vi "01_dosing.vi"() -> ()   [LabVIEW 2024]
panel:
  out "appended array":bool[](array[boolean])
  in  "Dispense Aliquot (Digital Output (0.4)":bool
  in  "Stop":bool
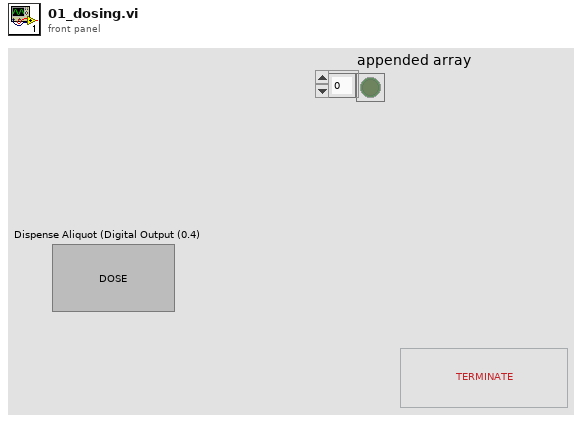
[diagram p1: front panel]
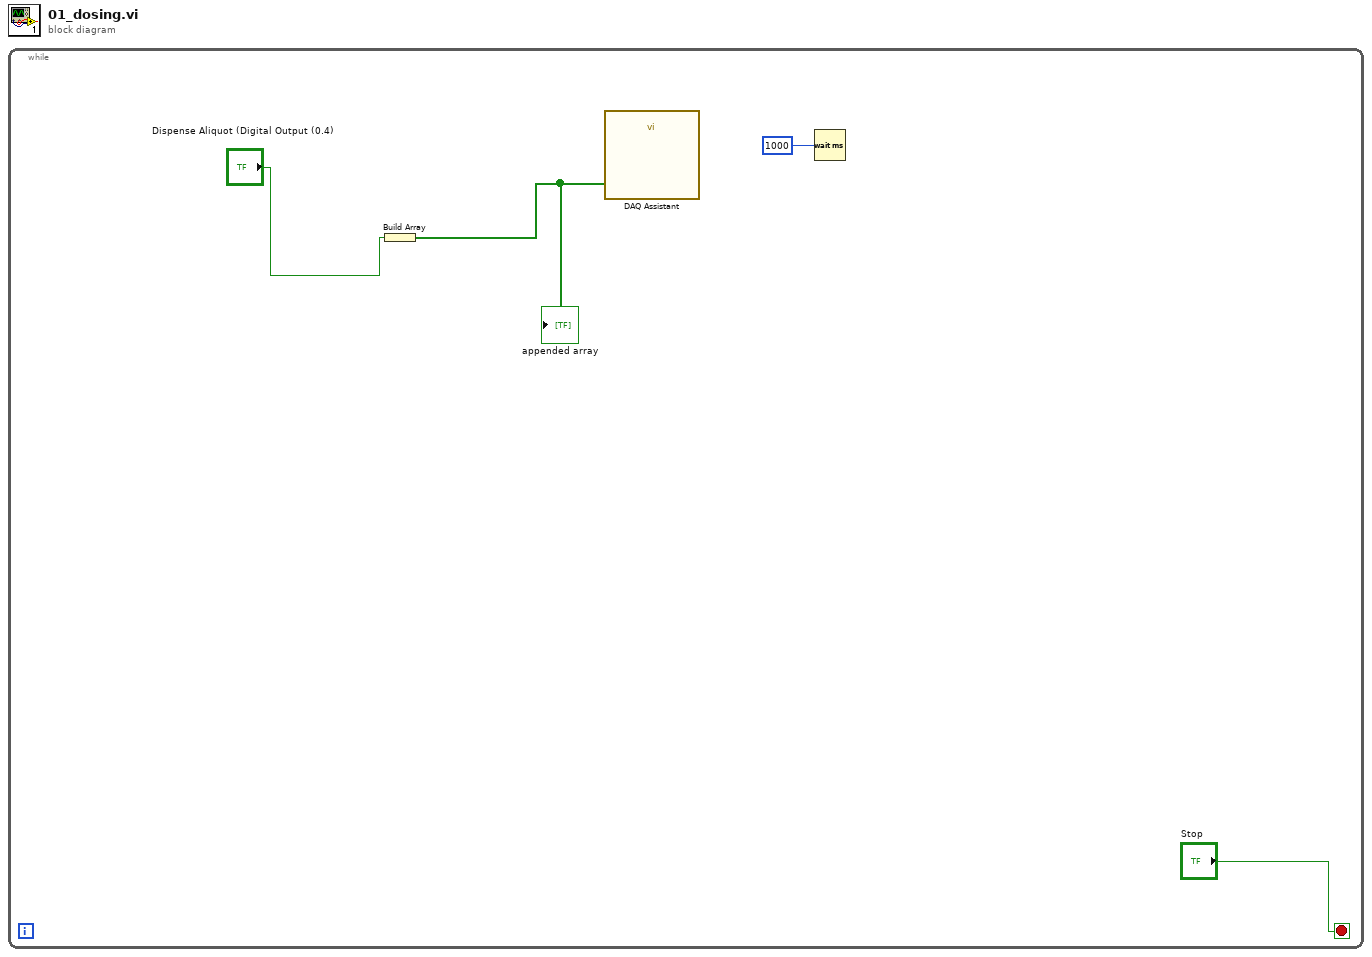
[diagram p0: block diagram]
diagram:
  n1 = while {
    stop <- "Stop" stop-if-true
    n2 = Build Array("Dispense Aliquot (Digital Output (0.4)") -> (w2:bool[])
    "appended array" <- w2
    n3 = call "DAQ Assistant"("data"=w2) -> ()  [unwired: 17 in, 2 out]
    n4 = Wait (ms)(milliseconds to wait=u32 1000 ("millisecond timer value")) -> ()  [unwired: 1 out]
  }
